vi "Init UI.vi"(8 "error in (no error)":errorcluster, 11 "View in":refnum<class "View.lvclass">) -> (0 "error out":errorcluster, 3 "View out":refnum<class "View.lvclass">)   [LabVIEW 2020, in "View.lvclass"]
uses:
  View.lvclass
  View.lvclass/View.ctl
  Controller/Controller.lvclass
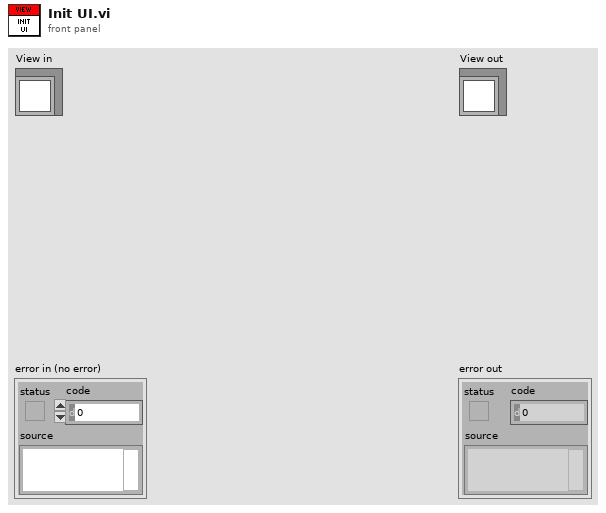
[diagram p1: front panel]
types:
  T1 = cluster{"View:Integer":refnum<vi>, "Model:Integer":refnum<vi>}
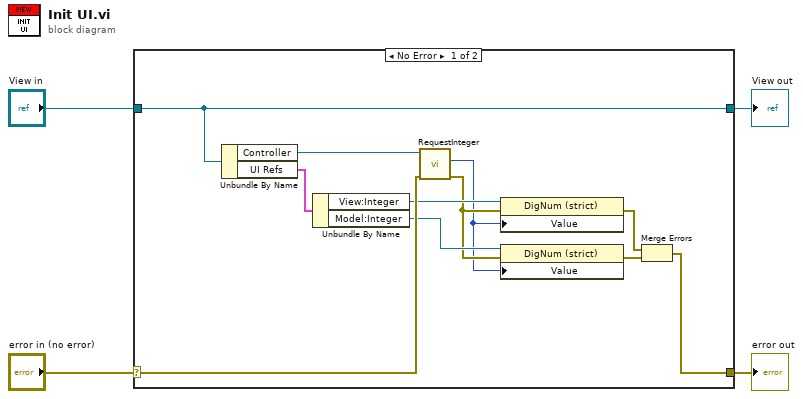
[diagram p0: block diagram]
diagram:
  n1 = case shown="No Error" "error in (no error)" {
    selector: "error in (no error)" -> [w13 w17]
    tunnel: [w5 w17] -> w3
    tunnel: [w15 w16] -> w1
    tunnel: "View in" -> [w15 w16]
    frame No Error {
      n2 = Unbundle By Name(w15) -> ("Controller"=w14:refnum<class "Controller.lvclass">, "UI Refs"=w12:T1)
      n3 = Unbundle By Name(w12) -> ("View:Integer"=w11:refnum<vi>, "Model:Integer"=w10:refnum<vi>)
      n4 = call "RequestInteger.vi"("error in (no error)"=w13, "Controller in"=w14) -> ("error out"=w9:errorcluster, "Integer"=w8:i32)  [unwired: 7 in, 1 out]
      n5 = property class="DigNum (strict)"(reference=w11, error in=w9, "Value"=w8) -> (error out=w7:errorcluster)  [unwired: 1 out]
      n6 = property class="DigNum (strict)"(reference=w10, error in=w9, "Value"=w8) -> (error out=w6:errorcluster)  [unwired: 1 out]
      n7 = Merge Errors(w7, w6) -> (w5:errorcluster)
    }
    frame Error {
    }
  }
  "error out" <- w3
  "View out" <- w1
